vi "Make_Tree_Item.vi"(8 "error in (no error)":errorcluster, 11 "IB_DotNET in":refnum<class "IB_DotNET.lvclass">) -> (0 "error out":errorcluster, 3 "TreeSrcItem":refnum<class "IB_Tree_Item_Source.lvclass">)   [LabVIEW 2020, in "IB_DotNET.lvclass"]
uses:
  <vilib>/AppBuilder/IB_Classes/Source/Container/Build/NET/IB_DotNET.lvclass
  <vilib>/AppBuilder/IB_Classes/Source/Container/Build/NET/IB_DotNET.lvclass/IB_DotNET.ctl
  <vilib>/AppBuilder/IB_Classes/Tree_Item_Source_NET/IB_Tree_Item_Source_DotNET.lvclass
  e:/builds/penguin/labview/branches/2020/dev/dist/vi.lib/AppBuilder/IB_Classes/Source/Container/Build/IB_Source_Build.lvclass
  e:/builds/penguin/labview/branches/2020/dev/dist/vi.lib/AppBuilder/IB_Classes/Source/Container/IB_Source_Container.lvclass
  e:/builds/penguin/labview/branches/2020/dev/dist/vi.lib/AppBuilder/IB_Classes/Source/IB_Source.lvclass
  e:/builds/penguin/labview/branches/2020/dev/dist/vi.lib/AppBuilder/IB_Classes/Source/Container/Build/NET/IB_DotNET.lvclass
  e:/builds/penguin/labview/branches/2020/dev/dist/vi.lib/AppBuilder/IB_Classes/Tree_Item_Source_Build/IB_Tree_Item_Source_Build.lvclass
  e:/builds/penguin/labview/branches/2020/dev/dist/vi.lib/AppBuilder/IB_Classes/Tree_Item_Source_Container/IB_Tree_Item_Source_Container.lvclass
  e:/builds/penguin/labview/branches/2020/dev/dist/vi.lib/AppBuilder/IB_Classes/Tree_Item_Source/IB_Tree_Item_Source.lvclass
  e:/builds/penguin/labview/branches/2020/dev/dist/vi.lib/AppBuilder/IB_Classes/Tree_Item/IB_Tree_Item.lvclass
  e:/builds/penguin/labview/branches/2020/dev/dist/vi.lib/AppBuilder/IB_Classes/Tree_Item_Source_NET/IB_Tree_Item_Source_DotNET.lvclass
  <vilib>/AppBuilder/IB_Classes/Tree_Item_Source/IB_Tree_Item_Source.lvclass
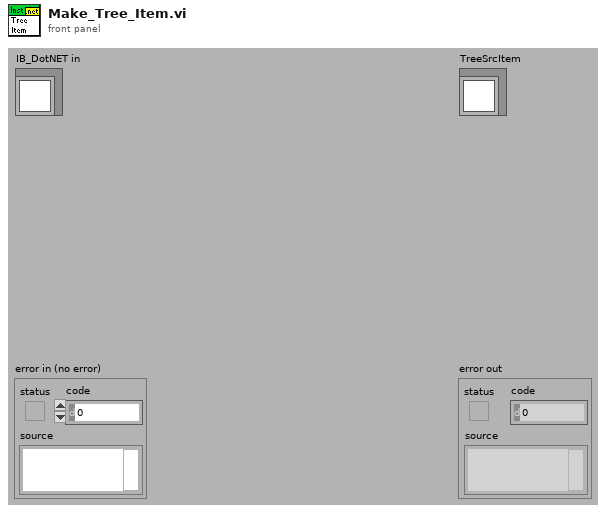
[diagram p1: front panel]
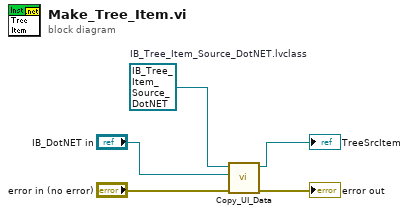
[diagram p0: block diagram]
diagram:
  w1 = refnum<class "IB_Tree_Item_Source_DotNET.lvclass"> refnum  # IB_Tree_Item_Source_DotNET.lvclass
  n1 = call-dynamic "Copy_UI_Data.vi"("error in (no error)"="error in (no error)", "IB_Source in"="IB_DotNET in", "IB_TreeContainerItem.lvclass"=w1) -> ("error out"=→"error out":errorcluster, "IB_TreeContainerItem out"=→"TreeSrcItem":refnum<class "IB_Tree_Item_Source_DotNET.lvclass">)  [unwired: 7 out]
